vi "Main_03a.vi"() -> ()   [LabVIEW 2020]
panel:
  out "Array":i32[](array[numeric])
  out "sum":i32
  in  "Example 2":string="dbcZDBCZ"
  out "unsigned byte array 2":u8[](array[numeric])
  out "unsigned byte array":u8[](array[numeric])
  in  "Puzzle":string="DsPhSBQQQhqmBDhPDsFwjwsLjlRjlttvjvvtRb\nrNJMNNbrHrtjHLHjvwtg\nfNbNzZdrZnMnMPnQShFPDmnqFm\nQWVCFfQffgQCVZzVVpHsHJBqtpspJFRHqq\nmwDbmnnGNlNcwNDDNRbnNDlJTpBJBtJGtPTLsBGqTqqsqp\nMlSdnScRnnmmDjSdNSdCzvggWzrgzjvfvrgVzW\ngsMljbrjlZlWcWMJrWwTwbmwQbmmLDQQLhwL\nCdgpzdgpgnfThHfFRwhfRf\nSptgpSpnCNpVSGNPvPGSddcMWjMrjqBsJcWqMcBWcVlZ\nJcJLQQFWhQJPJpWcwjHvMQvnnlMvzBHd\ntCtGZrmVRmVGTVTtCfRTCHHNNvdNzmdMvMlNzvwdvw\nCTGGRftfSGtGTGDLbFchSgSWWWcM\nQcMFQrvrQbvtczbVbjbMzZzRpqmDDmqqnNzCDCDC\nSHHfPJssGLPSdHThLhHdRmqNmNssnNmNCNnpjmsn\nLhLJfTdLJwfgPTdfGccrtjcMrccwvcrrFr\njFLLLqDGjbtqLCChpMMhMBvpwMTmffpZ\nZnJHRncHHgnrsrZffTdMdMBfmMvfvR\nN..."
  in  "Example":string="vJrwpWtwJgWrhcsFMMfFFhFp\njqHRNqRjqzjGDLGLrsFMfFZSrLrFZsSL\nPmmdzqPrVvPwwTWBwg\nwMqvLMZHhHMvwLHjbvcjnnSBnvTQFn\nttgJtRGJQctTZtZT\nCrZsJsPPZsGzwwsLwLmpwMDw"
  # "--- Day 3: Rucksack Reorganization ---\nOne Elf has the important job of loading all of the rucksacks with supplies for the jungle journey. Unfortunately, that Elf didn't quite follow the packing instructions, and so a few items now need to be rearranged.\n\nEach rucksack has two large compartments. All items of a given type are meant to go into exactly one of the two compartments. The Elf that did the packing failed to follow this rule for exactly one item type per rucksack.\n\nThe Elves have made a list of all of the items currently in each rucksack (your puzzle input), but they need your help finding the errors. Every item type is identified by a single lowercase or uppercase letter (that is, a and A refer to different types of items).\n\nThe list of items for each rucksack is given as characters all on a single line. A given rucksack always has the same number of items in each of its two compartments, so the first half of the characters represent items in the first compartment, while the second half of the characters represent items in the second compartment.\n\nFor example, suppose you have the following list of contents from six rucksacks:\n\nvJrwpWtwJgWrhcsFMMfFFhFp\njqHRNqRjqzjGDLGLrsFMfFZSrLrFZsSL\nPmmdzqPrVvPwwTWBwg\nwMqvLMZHhHMvwLHjbvcjnnSBnvTQFn\nttgJtRGJQctTZtZT\nCrZsJsPPZsGzwwsLwLmpwMDw\n\nThe first rucksack contains the items vJrwpWtwJgWrhcsFMMfFFhFp, which means its first compartment contains the items vJrwpWtwJgWr, while the second compartment contains the items hcsFMMfFFhFp. The only item type that appears in both compartments is lowercase p.\nThe second rucksack's compartments contain jqHRNqRjqzjGDLGL and rsFMfFZSrLrFZsSL. The only item type that appears in both compartments is uppercase L.\nThe third rucksack's compartments contain PmmdzqPrV and vPwwTWBwg; the only common item type is uppercase P.\nThe fourth rucksack's compartments only share item type v.\nThe fifth rucksack's compartments only share item type t.\nThe sixth rucksack's compartments only share item type s.\nTo help prioritize item rearrangement, every item type can be converted to a priority:\n\nLowercase item types a through z have priorities 1 through 26.\nUppercase item types A through Z have priorities 27 through 52.\nIn the above example, the priority of the item type that appears in both compartments of each rucksack is 16 (p), 38 (L), 42 (P), 22 (v), 20 (t), and 19 (s); the sum of these is 157.\n\nFind the item type that appears in both compartments of each rucksack. What is the sum of the priorities of those item types?"
  # "8176"
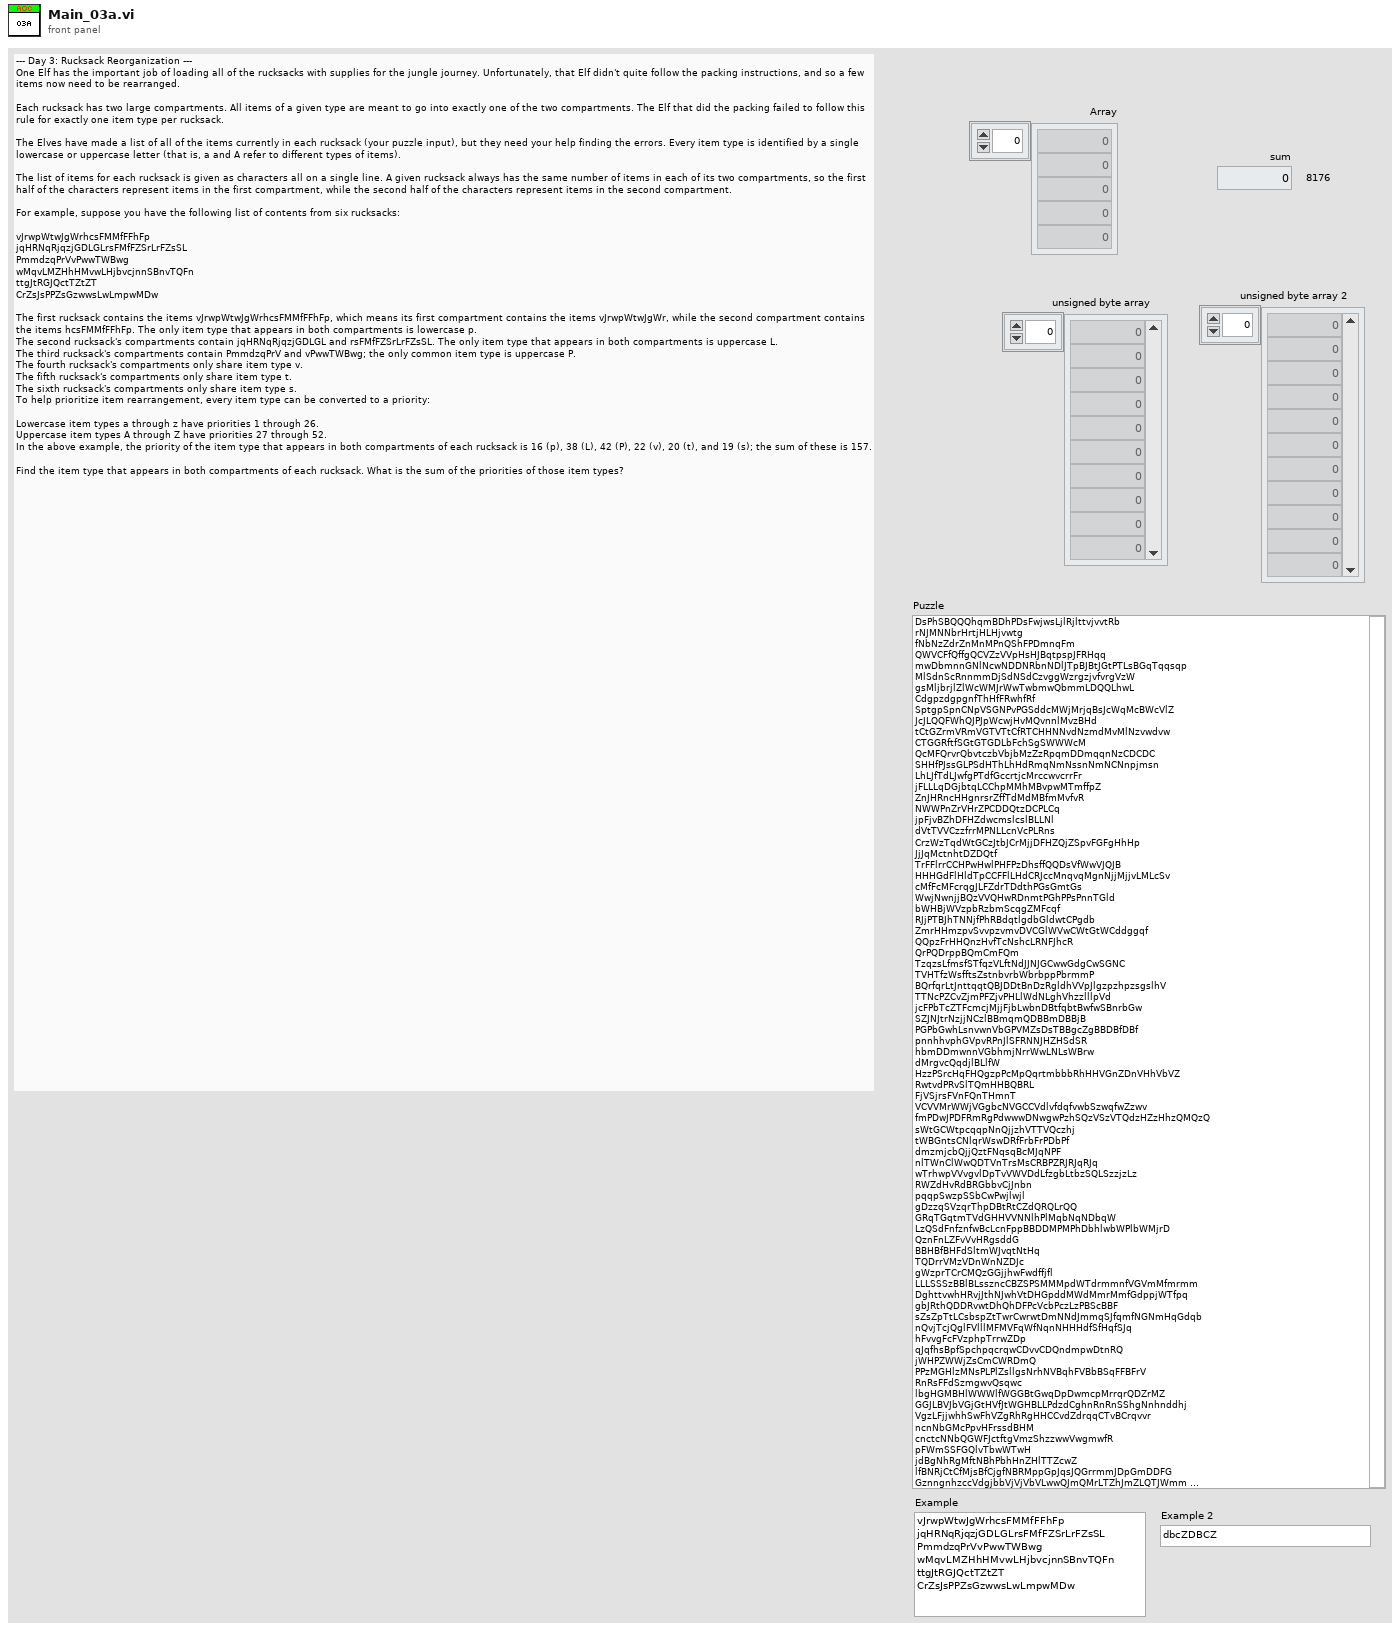
[diagram p1: front panel]
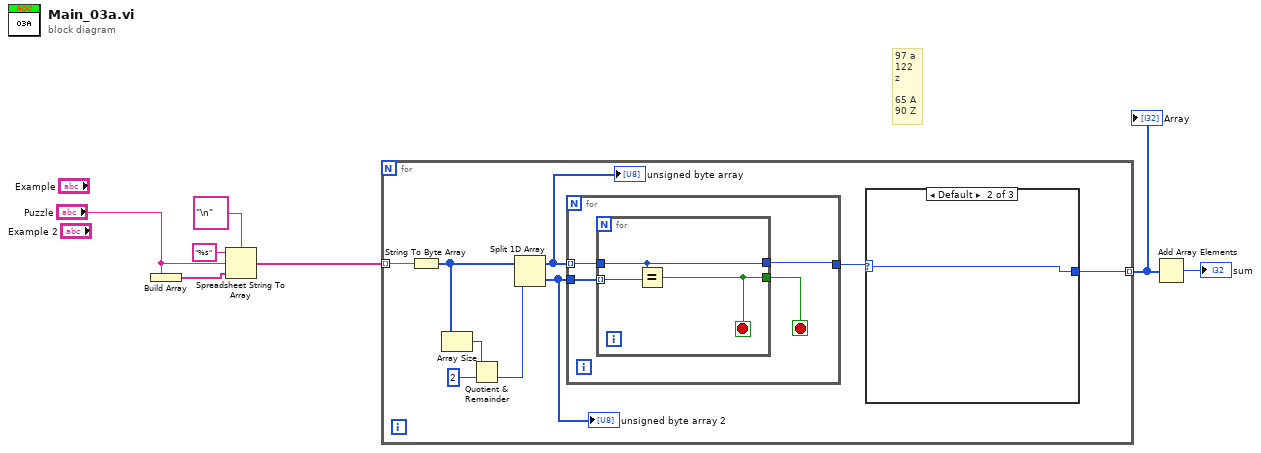
[diagram p0: block diagram]
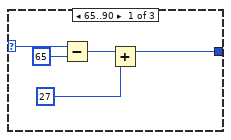
[diagram p2: hidden frame]
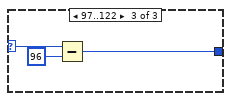
[diagram p3: hidden frame]
diagram:
  # "97 a\n122 z\n\n65 A\n90 Z"
  n1 = Build Array("Puzzle") -> (w7:string[])
  n2 = Spreadsheet String To Array(delimiter (Tab)="\n", format string="%s", spreadsheet string="Puzzle", array type (2D Dbl)=w7) -> (array=w4:string[])
  n3 = for {
    tunnel: w4 -> [w16] mode=indexing
    tunnel: [w8] -> w3 mode=indexing
    n4 = String To Byte Array(string=w16) -> (unsigned byte array=w12:u8[])
    n5 = Array Size(array=w12) -> (size(s)=w15:i32)
    n6 = Quotient & Remainder(x=w15, y=2) -> (floor(x/y)=w13:i32)  [unwired: 1 out]
    n7 = Split 1D Array(array=w12, index=w13) -> (first subarray=w11:u8[], second subarray=w10:u8[])
    "unsigned byte array" <- w11
    "unsigned byte array 2" <- w10
    n8 = for {
      tunnel: w11 -> [w28] mode=indexing
      tunnel: w10 -> [w29]
      tunnel: [w26] -> w9
      stop <- w27 stop-if-true
      n9 = for {
        tunnel: w29 -> [w32] mode=indexing
        tunnel: w28 -> [w31]
        tunnel: [w31] -> w26
        tunnel: [w30] -> w27
        stop <- w30 stop-if-true
        n10 = Equal?(x=w31, y=w32) -> (x = y?=w30:bool)
      }
    }
    n11 = case shown="Default" w9 {
      selector: w9 -> [w21 w22 w25]
      tunnel: [w19 w22 w23] -> w8
      frame 65..90 {
        n12 = Subtract(x=w21, y=u8 65) -> (x-y=w20:u8)
        n13 = Add(x=w20, y=27) -> (x+y=w19:i32)
      }
      frame Default {
      }
      frame 97..122 {
        n14 = Subtract(x=w25, y=u8 96) -> (x-y=w23:u8)
      }
    }
  }
  "Array" <- w3
  n15 = Add Array Elements(numeric array=w3) -> (sum=→"sum":i32)
